vi "Dead Zone.vi"   [LabVIEW 2017, in "NI_AdvCtrl_nonlinear.lvlib"]
doc: "LabVIEW no longer supports this VI. You can obtain similar functionality by installing the LabVIEW Simulation Module.\n\nRealizes a region of zero output, the so-called dead zone. The output is zero, if the inequalities start of dead zone < input < end of dead zone hold true."
uses:
  <vilib>/addons/control/advanced/NI_AdvCtrl_nonlinear.lvlib
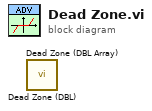
[diagram p0: block diagram]
diagram:
  n1 = call <vilib>:"Dead Zone (DBL).vi"() -> ()  [unwired: 4 in, 1 out]
  n2 = call <vilib>:"Dead Zone (DBL Array).vi"() -> ()  [unwired: 4 in, 1 out]
